vi "ADS1115-ADC16-bit-I2C-v2.vi"() -> ()   [LabVIEW 2014]
uses:
  <vilib>/MakerHub/LINX/Private/Local IO/LinxI2cWrite.vi
  <vilib>/MakerHub/LINX/Public/Utilities/Check Channel.vi
  <vilib>/MakerHub/LINX/Public/Utilities/Open Serial.vi
  <vilib>/MakerHub/LINX/Private/Utilties/Generate Error.vi
  <vilib>/MakerHub/LINX/LMH-LINX.lvlib
panel:
  out "Waveform Chart":sgl(graph)
  out "freq":dbl
  out "Magnetic Field (Oe)":sgl format="%#_5f"
  out "(hi.lo)":u16
  in  "millisecond multiple":u32
  out "Device Name":string
  out "Error Out":errorcluster
  in  "stop":bool
  in  "Serial Port":refnum<visa-resource-name>="N/A"
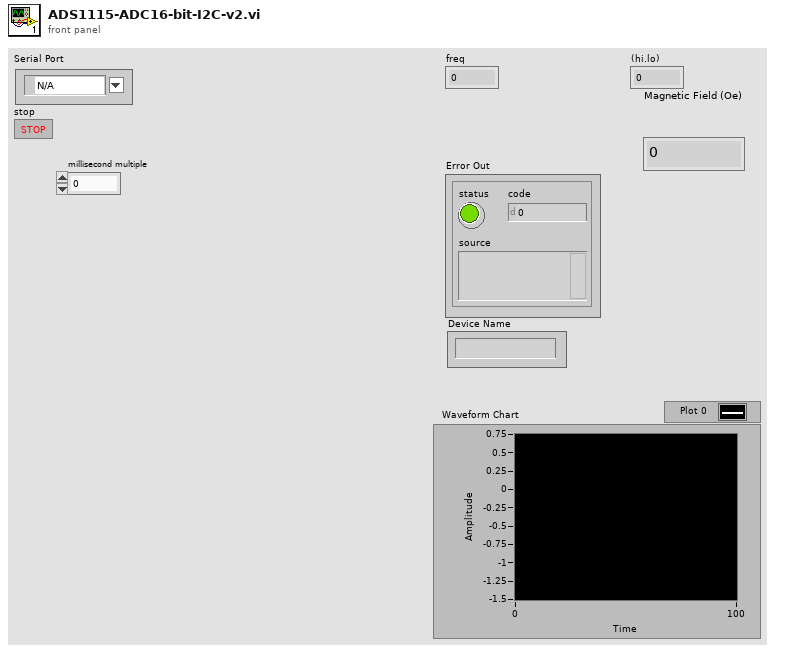
[diagram p1: front panel]
types:
  T1 = typedef "LMH-LINX.lvlib/LINX Ref.ctl" = cluster{"IO":T2, "Interface":T3, "LINX Device Config":T4}
  T2 = typedef "LMH-LINX.lvlib/Platform.ctl" = enum16{"Remote", "Local"}
  T3 = typedef "LMH-LINX.lvlib/Interface.ctl" = enum16{"Serial", "TCP"}
  T4 = typedef "LMH-LINX.lvlib/Device.lvlib/LINX Device Config.ctl" = cluster{"Interface":T3, "COM Port":refnum<visa-resource-name>, "TCP Configuration":T5, "Device Family":u8, "Device ID":u8, "Device Name":string, "TCP Ref":refnum<k5>, "Channels":T6}
  T5 = typedef "LMH-LINX.lvlib/Device.lvlib/TCP Config.ctl" = cluster{"IP Address":string, "Port":u16}
  T6 = typedef "LMH-LINX.lvlib/Channels.ctl" = cluster{"DI":u8[], "DO":u8[], "AI":u8[], "AO":u8[], "PWM":u8[], "QE":u8[], "UART":u8[], "I2C 2":u8[], "SPI":u8[], "CAN":u8[], "Servo":u8[], "AI Ref (V)":dbl, "AI Resolution (Bits)":u8, "AO Ref (V)":dbl, "AO Resolution (Bits)":u8}
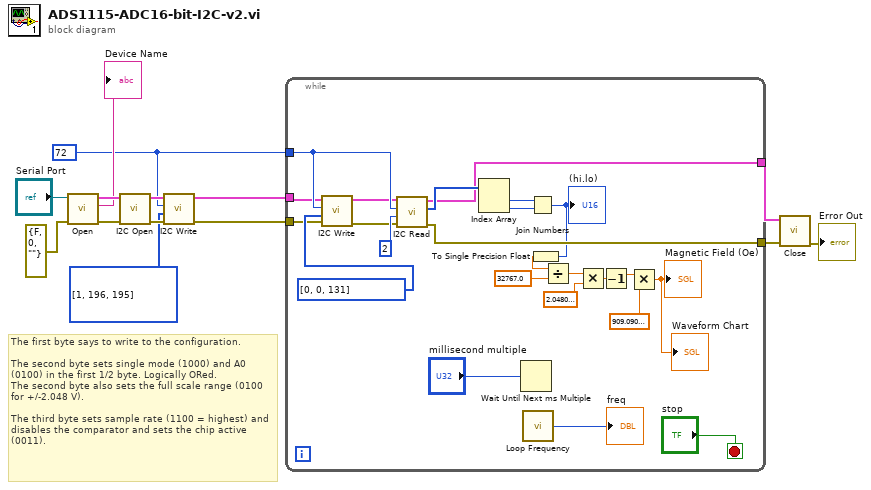
[diagram p0: block diagram]
diagram:
  w3 = 72
  # "The first byte says to write to the configuration.\n\nThe second byte sets single mode (1000) and A0 (0100) in the first 1/2 byte. Logically ORed.\nThe second byte also sets the full scale range (0100 for +/-2.048 V).\n\nThe third byte sets sample rate (1100 = highest) and disables the comparator and sets the chip active (0011)."
  n1 = call-poly <vilib>:"Open.vi"("Error In"=errorcluster {"status"=FALSE, "code"=0, "source"=""}, "Serial Port"="Serial Port") -> ("Error Out"=w12:errorcluster, "Device Name"=→"Device Name":string, "LINX Resource"=w11:T1)  [unwired: 7 in]
  n2 = call <vilib>:"I2C Open.vi"("Error In"=w12, "LINX Resource"=w11) -> ("Error Out"=w10:errorcluster, "LINX Resource"=w9:T1)  [unwired: 8 in]
  n3 = call <vilib>:"I2C Write.vi"("Error In"=w10, "Data"=u8[] [1, 196, 195], "I2C Slave Address (0)"=w3, "LINX Resource"=w9) -> ("Error Out"=w1:errorcluster, "LINX Resource"=w2:T1)  [unwired: 6 in]
  n4 = while {
    tunnel: w2 -> [w30]
    tunnel: w1 -> [w29]
    tunnel: w3 -> [w32]
    tunnel: [w35] -> w6
    tunnel: [w34] -> w4
    stop <- "stop" stop-if-true
    n5 = call <vilib>:"I2C Write.vi"("Error In"=w29, "Data"=u8[] [0, 0, 131], "I2C Slave Address (0)"=w32, "LINX Resource"=w30) -> ("Error Out"=w27:errorcluster, "LINX Resource"=w28:T1)  [unwired: 6 in]
    n6 = call <vilib>:"I2C Read.vi"("Error In"=w27, "Bytes To Read"=u8 2, "I2C Slave Address (0)"=w32, "LINX Resource"=w28) -> ("Error Out"=w35:errorcluster, "Data"=w36:u8[], "LINX Resource"=w34:T1)  [unwired: 5 in]
    n7 = Index Array(array=w36) -> (element #1=w24:u8, element #2=w23:u8)  [unwired: 2 in]
    n8 = Wait Until Next ms Multiple(millisecond multiple="millisecond multiple") -> ()  [unwired: 1 out]
    n9 = call <vilib>:"Loop Frequency.vi"() -> ("Loop Rate (Hz)"=→"freq":u32)
    n10 = Join Numbers(hi=w24, lo=w23) -> ((hi.lo)=w26:u16)
    "(hi.lo)" <- w26
    n11 = To Single Precision Float(number=w26) -> (single precision float=w19:sgl)
    n12 = Divide(x=w19, y=sgl 32767.0) -> (x/y=w22:sgl)
    n13 = Multiply(x=w22, y=sgl 2.048) -> (x*y=w21:sgl)
    n14 = Decrement(x=w21) -> (x-1=w16:sgl)
    n15 = Multiply(x=w16, y=sgl 909.09) -> (x*y=→"Magnetic Field (Oe)" →"Waveform Chart":sgl)
  }
  n16 = call <vilib>:"Close.vi"("Error In"=w6, "LINX Resource"=w4) -> ("Error Out"=→"Error Out":errorcluster)  [unwired: 9 in]
